vi "Write Required Absolute Epsilon.vi"(8 "error in (no error)":errorcluster, 10 "Required Absolute Epsilon":dbl=1e-06, 11 "FP Equal in":refnum<class "FP Equal.lvclass">) -> (0 "error out":errorcluster, 3 "FP Equal out":refnum<class "FP Equal.lvclass">)   [LabVIEW 2018, in "FP Equal.lvclass"]
uses:
  FP Equal.lvclass
  FP Equal.lvclass/FP Equal.ctl
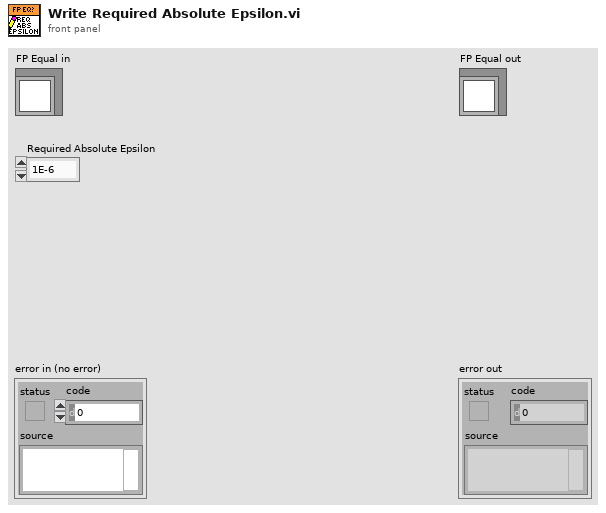
[diagram p1: front panel]
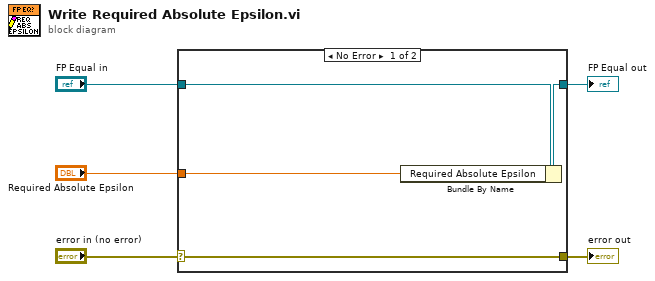
[diagram p0: block diagram]
diagram:
  n1 = case shown="No Error" "error in (no error)" {
    selector: "error in (no error)" -> [w9 w10]
    tunnel: [w9 w10] -> w4
    tunnel: [w7 w11] -> w2
    tunnel: "FP Equal in" -> [w8 w11]
    tunnel: "Required Absolute Epsilon" -> [w6 _]
    frame No Error {
      n2 = Bundle By Name(cluster=w8, "Required Absolute Epsilon"=w6) -> (w7:refnum<class "FP Equal.lvclass">)
    }
    frame Error {
    }
  }
  "error out" <- w4
  "FP Equal out" <- w2
